vi "UHR-Fleezers Control (host) - 11.9b.vi"() -> ()   [LabVIEW 2014] (continued)
        n1961 = Or(x="Move to Position 5", y="Lower Ch. Cap.") -> (x .or. y?=w2805:bool)
        n1962 = Build Array("Move to Position 1", "Move to Position 2", "Move to Position 3", "Move to Position 4", w2805) -> (w2808:bool[])
        n1963 = Boolean Array To Number(Boolean array=w2808) -> (number=w2807:u32)
        n1964 = Logarithm Base 2(1:w2807) -> (0:w2806:dbl)
        n1965 = flat-sequence {
          tunnel: w2806 -> [w2817]
          tunnel: w2803 -> [w2815]
          tunnel: w2802 -> [w2814]
          frame #0 {
            n1966 = local read "Saved Stage Positions"() -> (w2825:dbl[][])
            n1967 = Array Subset(array=w2825, index (row)=w2817, length (row)=1 ("length"), index (col)=1 ("index"), length (col)=3 ("length")) -> (w2822:dbl[][])
            n1968 = Reshape Array(w2822, 3 ("dimension size")) -> (w2820:dbl[])
            n1969 = Array To Cluster(array=w2820) -> (cluster=w2819:cluster{"[0]":dbl, "[1]":dbl, "[2]":dbl})
            n1970 = call "Set Stage Position.vi"("Position"=w2819, "error in"=w2814, "VISA resource name in"=w2815) -> ("error out"=w2818:errorcluster)  [unwired: 2 out]
            n1971 = local write "Stage Moving"(TRUE ("Stage Moving")) -> ()
            n1972 = local write "Stage Control Serial Error"(w2818) -> ()
          }
          frame #1 {
            n1973 = local write "Stage Moving"(FALSE ("Stage Moving")) -> ()
            n1974 = call <vilib>:"Beep.vi"() -> ()  [unwired: 3 in, 9 out]
          }
        }
      }
      event "Set Current\nPos to 0,0,0": Value Change {
        # "DH is \"Define Home\""
        n1975 = event-data() -> ()  [unwired: 1 in, 6 out]
        n1976 = local write "Set Current\nPos to 0,0,0"(FALSE ("Set Current\nPos to 0,0,0")) -> ()
        n1977 = Concatenate Strings("1DH" ("string"), ";" ("string"), "2DH" ("string"), ";" ("string"), "3DH" ("string"), "\r") -> (w2833:string)
        n1978 = call-poly "VISA Configure Serial Port"("VISA resource name"=w2838, "baud rate (9600)"=u32 19200, "error in (no error)"=w2837) -> ("VISA resource name out"=w2835:refnum<visa-resource-name>, "error out"=w2834:errorcluster)  [unwired: 11 in]
        n1979 = VISA Write(VISA resource name=w2835, write buffer=w2833, error in (no error)=w2834) -> (error out=w2828:errorcluster)  [unwired: 2 out]
        n1980 = local write "Stage Control Serial Error"(w2828) -> ()
      }
      event "Got ADig bead": Value Change {
        n1981 = event-data() -> ()  [unwired: 1 in, 5 out]
        n1982 = flat-sequence {
          frame #0 {
            n1983 = local read "Cap 1 Samp Flow ON"() -> (w2843:bool)
            n1984 = case shown="True" w2843 {
              frame False {
              }
              frame True {
                n1985 = property on="Sample Channel\nFlow" class="Bool (strict)"("Val(Sgnl)"=TRUE ("Value (Signaling)")) -> ()  [unwired: 2 in, 2 out]
              }
            }
          }
          frame #1 {
            n1986 = property on="Inject Pump 3" class="Bool (strict)"("Val(Sgnl)"=FALSE ("Value (Signaling)")) -> ()  [unwired: 2 in, 2 out]
            n1987 = local write "Target"(FALSE ("Target")) -> ()
          }
          frame #2 {
            n1988 = property on="Move Cap. 1 (DNA Bottom)" class="Bool (strict)"("Val(Sgnl)"=TRUE ("Value (Signaling)")) -> ()  [unwired: 2 in, 2 out]
          }
        }
      }
      event "Force FB Script": Value Change {
        n1989 = event-data() -> ()  [unwired: 1 in, 5 out]
        n1990 = local write "Force FB Script"(FALSE ("Force FB Data\nScript")) -> ()
        n1991 = flat-sequence {
          tunnel: w2854 -> [w2858]
          tunnel: w2855 -> [w2859]
          tunnel: [w2859] -> w2850
          tunnel: [w2858] -> w2849
          tunnel: w2850 -> [w2862]
          tunnel: w2849 -> [w2861]
          tunnel: ["Trap Trig Fl."] -> w2851
          tunnel: [w2904] -> w2852
          tunnel: w2851 -> [w2904]
          tunnel: [w2908] -> w2853
          tunnel: w2852 -> [w2908]
          tunnel: w2853 -> [w2910]
          frame #0 {
            n1992 = property on="Trap D (MHz)" class="DigNum (strict)"("Val(Sgnl)"="Trap D Before Moving") -> ()  [unwired: 2 in, 2 out]
          }
          frame #1 {
            n1993 = local read "Saved Stage Positions"() -> (w2864:dbl[][])
            n1994 = local write "FB Trap Pos Offset"(0.0 ("FB Trap Pos Offset")) -> ()
            n1995 = property on="Trap Pos. FB Offset Factor" class="DigNum (strict)"("Val(Sgnl)"=i64 0 ("Value (Signaling)")) -> ()  [unwired: 2 in, 2 out]
            n1996 = local write "Stage Moving"(TRUE ("Stage Moving")) -> ()
            n1997 = call "move to saved stage position.vi"("error in"=w2861, "Stage VISA resource name in"=w2862, "Position"="Stage Position To Establish FB", "Saved Stage Positions"=w2864) -> ("error out"=w2860:errorcluster)  [unwired: 1 out]
            n1998 = local write "Stage Control Serial Error"(w2860) -> ()
          }
          frame #2 {
            n1999 = call <vilib>:"Beep.vi"("duration (msec)"=u32 100, "frequency (Hz)"=u32 20) -> ()  [unwired: 1 in, 9 out]
            n2000 = local write "Stage Moving"(FALSE ("Stage Moving")) -> ()
            n2001 = property on="Tab Control 2" class="TabCtl (strict)"("Val(Sgnl)"=T6."Feedback on Trap Position" ("Value (Signaling)")) -> ()  [unwired: 2 in, 2 out]
            n2002 = stacked-sequence {
              frame #0 {
                n2003 = Multiply(x="Wait (s)", y=u32 1000 ("milliseconds to wait")) -> (x*y=w2873:u32)
                n2004 = property on="Trap D (MHz)" class="DigNum (strict)"("Val(Sgnl)"="Starting Trap D (MHz)") -> ()  [unwired: 2 in, 2 out]
                n2005 = Wait (ms)(milliseconds to wait=w2873) -> ()  [unwired: 1 out]
              }
              frame #1 {
                n2006 = property on="Set Reading to\nSetpoint" class="Bool (strict)"("Val(Sgnl)"=TRUE ("Value (Signaling)")) -> ()  [unwired: 2 in, 2 out]
              }
            }
            n2007 = property on="Tab Control" class="TabCtl (strict)"("Val(Sgnl)"=T4."Trap Control (RF)" ("Value (Signaling)")) -> ()  [unwired: 2 in, 2 out]
          }
          frame #3 {
            n2008 = Wait (ms)(milliseconds to wait=u32 500) -> ()  [unwired: 1 out]
          }
          frame #4 {
            n2009 = property on="Trap Pos. FB ON" class="Bool (strict)"("Val(Sgnl)"=TRUE ("Value (Signaling)")) -> ()  [unwired: 2 in, 2 out]
            n2010 = Wait (ms)(milliseconds to wait=u32 250) -> ()  [unwired: 1 out]
          }
          frame #5 {
            n2011 = case shown="\"1\"" "Remove Action Offset Dropdown" {
              tunnel: TRUE ("Value (Signaling)") -> [w2885 w2893 w2901]
              frame "1" {
                n2012 = flat-sequence {
                  tunnel: w2885 -> [w2892]
                  frame #0 {
                    n2013 = local read "factor"() -> (w2887:dbl)
                    n2014 = Greater Than 0?(x=w2887) -> (x > 0?=w2891:bool)
                    n2015 = Select(t=1.0, s=w2891, f=-1.0) -> (s? t:f=w2888:dbl)
                    n2016 = Multiply(x=w2888, y=w2887) -> (x*y=w2886:dbl)
                    n2017 = local write "factor"(w2886) -> ()
                  }
                  frame #1 {
                    n2018 = property on="Remove Offset to factor" class="Bool (strict)"("Val(Sgnl)"=w2892) -> ()  [unwired: 2 in, 2 out]
                  }
                }
              }
              frame "2" {
                n2019 = flat-sequence {
                  tunnel: w2893 -> [w2900]
                  frame #0 {
                    n2020 = local read "factor"() -> (w2894:dbl)
                    n2021 = Greater Than 0?(x=w2894) -> (x > 0?=w2899:bool)
                    n2022 = Select(t=-1.0, s=w2899, f=1.0) -> (s? t:f=w2897:dbl)
                    n2023 = Multiply(x=w2894, y=w2897) -> (x*y=w2896:dbl)
                    n2024 = local write "factor"(w2896) -> ()
                  }
                  frame #1 {
                    n2025 = property on="Remove Offset to factor" class="Bool (strict)"("Val(Sgnl)"=w2900) -> ()  [unwired: 2 in, 2 out]
                  }
                }
              }
              frame "0", Default {
                n2026 = property on="Remove Action Offset" class="Bool (strict)"("Val(Sgnl)"=w2901) -> ()  [unwired: 2 in, 2 out]
              }
            }
            n2027 = case shown="False" "Trap Trig Fl." {
              frame False {
                n2028 = case shown="True" "Green ON after FB ON?" {
                  selector: "Green ON after FB ON?" -> [_ w2903]
                  frame False {
                  }
                  frame True {
                    n2029 = property on="Green ON/Interlacing" class="Bool (strict)"("Val(Sgnl)"=w2903) -> ()  [unwired: 2 in, 2 out]
                  }
                }
              }
              frame True {
              }
            }
            n2030 = Wait (ms)(milliseconds to wait=u32 250) -> ()  [unwired: 1 out]
          }
          frame #6 {
            n2031 = property on="Start Saving" class="Bool (strict)"("Val(Sgnl)"=TRUE ("Value (Signaling)")) -> ()  [unwired: 2 in, 2 out]
            n2032 = Wait (ms)(milliseconds to wait=u32 5000) -> ()  [unwired: 1 out]
          }
          frame #7 {
            w2907 = TRUE ("Value (Signaling)")
            n2033 = property on="Rem fb disp offset" class="Bool (strict)"("Val(Sgnl)"=w2907) -> ()  [unwired: 2 in, 2 out]
            n2034 = property on="Remove Offset" class="Bool (strict)"("Val(Sgnl)"=w2907) -> ()  [unwired: 2 in, 2 out]
            n2035 = Wait (ms)(milliseconds to wait=u32 100) -> ()  [unwired: 1 out]
          }
          frame #8 {
            n2036 = case shown="True" w2910 {
              frame False {
              }
              frame True {
                n2037 = local write "Trap Trig. Fl."(TRUE ("Value (Signaling)")) -> ()
              }
            }
          }
          frame #9 {
            n2038 = local read "Tether"() -> (w2913:bool)
            n2039 = And(x="Start dipping after?", y=w2913) -> (x .and. y?=w2912:bool)
            n2040 = case shown="True" w2912 {
              frame False {
              }
              frame True {
                n2041 = flat-sequence {
                  frame #0 {
                    n2042 = Multiply(x="Delay before dipping (s)", y=1000.0) -> (x*y=w2916:dbl)
                    n2043 = Wait (ms)(milliseconds to wait=w2916) -> ()  [unwired: 1 out]
                  }
                  frame #1 {
                    n2044 = property on="Dip for Protein" class="Bool (strict)"("Val(Sgnl)"=TRUE ("Value (Signaling)")) -> ()  [unwired: 2 in, 2 out]
                    n2045 = local write "Scripts"(T29."Dipping") -> ()
                  }
                }
              }
            }
          }
        }
      }
      event "Rupture Script": Value Change {
        n2046 = event-data() -> ()  [unwired: 1 in, 5 out]
        n2047 = local write "Rupture Script"(FALSE ("Rupture Script")) -> ()
        n2048 = flat-sequence {
          frame #0 {
            w2922 = TRUE
            w2927 = FALSE
            # "Number 6 for now is the\nrupture-experiment\nparameters."
            n2049 = local read "Starting Trap D (MHz)"() -> (w2928:dbl)
            n2050 = local write "Restart DMA? (AOD)"(w2927) -> ()
            n2051 = Replace Array Subset(array=u32[] [0] ("Index Values"), new element=6, index=0) -> (w2923:u32[])
            n2052 = local write "Save scans"(w2927) -> ()
            n2053 = property on="Trap D (MHz)" class="DigNum (strict)"("Val(Sgnl)"=w2928) -> ()  [unwired: 2 in, 2 out]
            n2054 = property on="Saved AOD Raster Scan Parameter Sets" class="Arr (strict)"("Index Values"=w2923) -> ()  [unwired: 2 in, 2 out]
            n2055 = property on="Start Saving" class="Bool (strict)"("Val(Sgnl)"=w2922) -> ()  [unwired: 2 in, 2 out]
            n2056 = property on="Green ON/Interlacing" class="Bool (strict)"("Val(Sgnl)"=w2922) -> ()  [unwired: 2 in, 2 out]
          }
          frame #1 {
            n2057 = property on="Load parameters" class="Bool (strict)"("Val(Sgnl)"=TRUE ("Value (Signaling)")) -> ()  [unwired: 2 in, 2 out]
          }
        }
      }
      event "Fixed Traps Script": Value Change {
        n2058 = event-data() -> ()  [unwired: 1 in, 5 out]
        n2059 = local write "Fixed Traps Script"(FALSE ("Fixed Traps Data\nScript")) -> ()
        n2060 = flat-sequence {
          frame #0 {
            n2061 = case shown="True" "Green ON" {
              frame False {
              }
              frame True {
                n2062 = property on="Green ON/Interlacing" class="Bool (strict)"("Val(Sgnl)"=TRUE) -> ()  [unwired: 2 in, 2 out]
              }
            }
            n2063 = local write "Offset (nm)"(0.0 ("Offset (nm)")) -> ()
            n2064 = property on="Sample Channel\nFlow" class="Bool (strict)"("Val(Sgnl)"=FALSE ("Value (Signaling)")) -> ()  [unwired: 2 in, 2 out]
            n2065 = property on="Trap D (MHz)" class="DigNum (strict)"("Val(Sgnl)"="Fixed Traps Trap Delta (MHz)") -> ()  [unwired: 2 in, 2 out]
          }
          frame #1 {
            n2066 = Wait (ms)(milliseconds to wait=u32 1000) -> ()  [unwired: 1 out]
          }
          frame #2 {
            n2067 = local write "Start Saving"(TRUE ("Start Saving")) -> ()
          }
          frame #3 {
            n2068 = local read "Bead Sep. Int. Time (s)"() -> (w2938:dbl)
            n2069 = Multiply(x=w2938, y=1000.0) -> (x*y=w2940:dbl)
            n2070 = Wait (ms)(milliseconds to wait=w2940) -> ()  [unwired: 1 out]
          }
          frame #4 {
            n2071 = property on="Remove Offset" class="Bool (strict)"("Val(Sgnl)"=TRUE ("Value (Signaling)")) -> ()  [unwired: 2 in, 2 out]
          }
          frame #5 {
            n2072 = property on="Dip for Protein" class="Bool (strict)"("Val(Sgnl)"="Start dipping after?") -> ()  [unwired: 2 in, 2 out]
          }
        }
      }
      event "Got DNA bead": Value Change {
        n2073 = event-data() -> ()  [unwired: 1 in, 5 out]
        n2074 = flat-sequence {
          frame #0 {
            n2075 = local read "Daq spot flow on"() -> (w2945:bool)
            n2076 = case shown="True" w2945 {
              frame False {
              }
              frame True {
                n2077 = property on="Sample Channel\nFlow" class="Bool (strict)"("Val(Sgnl)"=TRUE ("Value (Signaling)")) -> ()  [unwired: 2 in, 2 out]
              }
            }
            n2078 = property on="Got DNA bead" class="Bool"("Key Focus"=FALSE) -> ()  [unwired: 2 in, 2 out]
          }
          frame #1 {
            n2079 = property on="Inject Pump 1" class="Bool (strict)"("Val(Sgnl)"=FALSE ("Value (Signaling)")) -> ()  [unwired: 2 in, 2 out]
          }
          frame #2 {
            n2080 = property on="Cal/Data Acq. Spot" class="Bool (strict)"("Val(Sgnl)"=TRUE ("Value (Signaling)")) -> ()  [unwired: 2 in, 2 out]
          }
        }
      }
      event "Take Stepping Data": Value Change {
        n2081 = event-data() -> ()  [unwired: 1 in, 5 out]
        n2082 = local read "Save ave N"() -> (w2957:dbl)
        n2083 = flat-sequence {
          tunnel: w2957 -> [w2959]
          tunnel: [w2959] -> w2952
          tunnel: [w2961] -> w2953
          tunnel: w2952 -> [w2961]
          tunnel: [w2963] -> w2954
          tunnel: w2953 -> [w2963]
          tunnel: [w2966] -> w2955
          tunnel: w2954 -> [w2966]
          tunnel: [w2968] -> w2956
          tunnel: w2955 -> [w2968]
          tunnel: [w2970] -> w2950
          tunnel: w2956 -> [w2970]
          tunnel: w2950 -> [w2973]
          tunnel: [w2973] -> w2949
          tunnel: w2949 -> [w2974]
          tunnel: [w2974] -> w2951
          tunnel: w2951 -> [w2980]
          frame #0 {
            n2084 = property on="Save ave N" class="DigNum (strict)"("Val(Sgnl)"="Save ave factor") -> ()  [unwired: 2 in, 2 out]
          }
          frame #1 {
            n2085 = Wait (ms)(milliseconds to wait=u32 100) -> ()  [unwired: 1 out]
          }
          frame #2 {
            n2086 = local read "Offset 2 Start (MHz)"() -> (w2965:dbl)
            n2087 = property on="Saved AOD Raster Scan Parameter Sets" class="Arr (strict)"("Index Values"=u32[] [2]) -> ()  [unwired: 2 in, 2 out]
            n2088 = property on="Trap D (MHz)" class="DigNum (strict)"("Val(Sgnl)"=w2965) -> ()  [unwired: 2 in, 2 out]
          }
          frame #3 {
            n2089 = property on="Load parameters" class="Bool (strict)"("Val(Sgnl)"=TRUE ("Value (Signaling)")) -> ()  [unwired: 2 in, 2 out]
          }
          frame #4 {
            n2090 = Wait (ms)(milliseconds to wait=u32 100) -> ()  [unwired: 1 out]
          }
          frame #5 {
            n2091 = property on="Trap Raster Scan" class="Bool (strict)"("Val(Sgnl)"=TRUE ("Value (Signaling)")) -> ()  [unwired: 2 in, 2 out]
          }
          frame #6 {
            n2092 = Wait (ms)(milliseconds to wait=u32 1000) -> ()  [unwired: 1 out]
          }
          frame #7 {
            n2093 = while {
              stop <- w2977 stop-if-true
              n2094 = local read "Raster Scanning..."() -> (w2979:bool)
              n2095 = local read "Saving..."() -> (w2978:bool)
              n2096 = Not(x=w2978) -> (.not. x?=w2975:bool)
              n2097 = Not(x=w2979) -> (.not. x?=w2976:bool)
              n2098 = And(x=w2976, y=w2975) -> (x .and. y?=w2977:bool)
            }
          }
          frame #8 {
            n2099 = property on="Save ave N" class="DigNum (strict)"("Val(Sgnl)"=w2980) -> ()  [unwired: 2 in, 2 out]
          }
        }
      }
      event "Step Size (nm)": Value Change {
        n2100 = event-data() -> ()  [unwired: 1 in, 5 out]
        n2101 = flat-sequence {
          frame #0 {
            n2102 = property on="Saved AOD Raster Scan Parameter Sets" class="Arr (strict)"("Index Values"=u32[] [1]) -> ()  [unwired: 2 in, 2 out]
          }
          frame #1 {
            n2103 = Multiply(x="N Steps", y="Step Size (nm)") -> (x*y=w2982:dbl)
            n2104 = property on="Scan Speed AOD (nm/s) 2" class="DigNum (strict)"("Value"="Step Size (nm)") -> ()  [unwired: 2 in, 2 out]
            n2105 = property on="Step Size AOD (nm) 2" class="DigNum (strict)"("Value"="Step Size (nm)") -> ()  [unwired: 2 in, 2 out]
            n2106 = property on="Scan Range AOD (nm) 2" class="DigNum (strict)"("Value"=w2982) -> ()  [unwired: 2 in, 2 out]
          }
        }
      }
      event "Take Detection Laser\nImage": Value Change {
        n2107 = event-data() -> ()  [unwired: 1 in, 5 out]
        n2108 = flat-sequence {
          tunnel: [w3010] -> w3000
          tunnel: [w3009] -> w2993
          tunnel: [w3008] -> w2985
          tunnel: [w3013] -> w3001
          tunnel: w3000 -> [w3013]
          tunnel: [w3012] -> w2994
          tunnel: w2993 -> [w3012]
          tunnel: [w3011] -> w2986
          tunnel: w2985 -> [w3011]
          tunnel: [w3017] -> w3002
          tunnel: w3001 -> [w3017]
          tunnel: [w3016] -> w2995
          tunnel: w2994 -> [w3016]
          tunnel: [w3015] -> w2987
          tunnel: w2986 -> [w3015]
          tunnel: [w3023] -> w3003
          tunnel: w3002 -> [w3023]
          tunnel: [w3022] -> w2996
          tunnel: w2995 -> [w3022]
          tunnel: [w3021] -> w2988
          tunnel: w2987 -> [w3021]
          tunnel: [w3027] -> w3004
          tunnel: w3003 -> [w3027]
          tunnel: [w3026] -> w2997
          tunnel: w2996 -> [w3026]
          tunnel: [w3025] -> w2989
          tunnel: w2988 -> [w3025]
          tunnel: [w3031] -> w3005
          tunnel: w3004 -> [w3031]
          tunnel: [w3030] -> w2998
          tunnel: w2997 -> [w3030]
          tunnel: [w3029] -> w2990
          tunnel: w2989 -> [w3029]
          tunnel: [w3035] -> w3006
          tunnel: w3005 -> [w3035]
          tunnel: [w3034] -> w2999
          tunnel: w2998 -> [w3034]
          tunnel: [w3033] -> w2991
          tunnel: w2990 -> [w3033]
          tunnel: w3006 -> [w3041]
          tunnel: w2999 -> [w3040]
          tunnel: [w3038] -> w2992
          tunnel: w2991 -> [w3038]
          tunnel: w2992 -> [w3042]
          frame #0 {
            n2109 = local read "Green ON/Interlacing"() -> (w3010:bool)
            n2110 = local read "Green laser mode"() -> (w3009:enum32{"Laser ON", "Laser OFF", "Interlace"})
            n2111 = local read "Green FB On/Off"() -> (w3008:bool)
          }
          frame #1 {
            n2112 = property on="Green FB On/Off" class="Bool (strict)"("Val(Sgnl)"=FALSE ("Value (Signaling)")) -> ()  [unwired: 2 in, 2 out]
          }
          frame #2 {
            n2113 = property on="Green ON/Interlacing" class="Bool (strict)"("Val(Sgnl)"=TRUE ("Value (Signaling)")) -> ()  [unwired: 2 in, 2 out]
            n2114 = property on="Flip Green Filter" class="Bool (strict)"("Val(Sgnl)"=TRUE ("Value (Signaling)")) -> ()  [unwired: 2 in, 2 out]
            n2115 = property on="Green laser mode" class="RadioBtnsControl (strict)"("Val(Sgnl)"=enum32{"Laser ON", "Laser OFF", "Interlace"}."Laser ON" ("Value (Signaling)")) -> ()  [unwired: 2 in, 2 out]
          }
          frame #3 {
            n2116 = Wait (ms)(milliseconds to wait=u32 500) -> ()  [unwired: 1 out]
          }
          frame #4 {
            n2117 = property on="Confocal\nImage" class="Bool (strict)"("Val(Sgnl)"=TRUE ("Value (Signaling)")) -> ()  [unwired: 2 in, 2 out]
          }
          frame #5 {
            n2118 = Wait (ms)(milliseconds to wait=u32 2000) -> ()  [unwired: 1 out]
          }
          frame #6 {
            n2119 = while {
              stop <- w3036 stop-if-true
              n2120 = local read "Saving..."() -> (w3037:bool)
              n2121 = Not(x=w3037) -> (.not. x?=w3036:bool)
            }
          }
          frame #7 {
            n2122 = property on="Flip Green Filter" class="Bool (strict)"("Val(Sgnl)"=TRUE ("Value (Signaling)")) -> ()  [unwired: 2 in, 2 out]
            n2123 = property on="Green ON/Interlacing" class="Bool (strict)"("Val(Sgnl)"=w3041) -> ()  [unwired: 2 in, 2 out]
            n2124 = property on="Green laser mode" class="RadioBtnsControl (strict)"("Val(Sgnl)"=w3040) -> ()  [unwired: 2 in, 2 out]
          }
          frame #8 {
            n2125 = property on="Green FB On/Off" class="Bool (strict)"("Val(Sgnl)"=w3042) -> ()  [unwired: 2 in, 2 out]
          }
        }
      }
      event "Stop All": Value Change {
        n2126 = event-data() -> ()  [unwired: 1 in, 5 out]
        n2127 = local read "Stop All"() -> (w3043:bool)
      }
    }
    n2128 = node-c288() -> ()  [unwired: 1 in, 1 out]
  }
  n2129 = node-c288() -> (w115:T21)  [unwired: 4 out]
  n2130 = timed-loop "Mouse control: trap position (AOM deflection), set confocal spot from image" {
    tunnel: [w3045] -> w203
    tunnel: w23 -> [w3044]
    timing: w115 -> [_]
    timing-out: [_] -> w114
    stop <- w3045 stop-if-true
    n2131 = node-c288() -> ()  [unwired: 2 out]
    n2132 = event shown="[0] \"Pane\": Mouse Down" {
      selector: _ -> [_ _]
      dyn-events: _ -> [_ _]
      timeout: _ -> [_ _]
      tunnel: w3044 -> [w3048 _]
      event Mouse Down {
        n2133 = event-data() -> ("Time"=w3050:u32, "Coords"=w3049:T7, "Button"=w3051:u16)  [unwired: 6 out]
        n2134 = case shown="1" w3051 {
          tunnel: w3050 -> [_ _ w3190]
          tunnel: w3049 -> [_ w3056 w3188]
          tunnel: w3048 -> [_ _ w3186]
          frame 0, Default {
          }
          frame 1 {
            n2135 = property on="APD 2" class="ImageControl"() -> ("Displayed Image Position"=w3070:cluster{"Left":i32, "Top":i32})  [unwired: 2 in, 2 out]
            n2136 = control-ref of="Primary Video Display"() -> (w3063:refnum<vi>)
            n2137 = property on="APD 1" class="ImageControl"() -> ("Displayed Image Position"=w3099:cluster{"Left":i32, "Top":i32})  [unwired: 2 in, 2 out]
            n2138 = property on="Detection Laser X" class="ImageControl"() -> ("Displayed Image Position"=w3096:cluster{"Left":i32, "Top":i32})  [unwired: 2 in, 2 out]
            n2139 = property on="Detection Laser Y" class="ImageControl"() -> ("Displayed Image Position"=w3095:cluster{"Left":i32, "Top":i32})  [unwired: 2 in, 2 out]
            n2140 = property on="APD 2" class="ImageControl"() -> ("Displayed Image Size"=w3069:cluster{"Width":u32, "Height":u32})  [unwired: 2 in, 2 out]
            n2141 = property on="APD 1" class="ImageControl"() -> ("Displayed Image Size"=w3097:cluster{"Width":u32, "Height":u32})  [unwired: 2 in, 2 out]
            n2142 = property on="Detection Laser X" class="ImageControl"() -> ("Displayed Image Size"=w3098:cluster{"Width":u32, "Height":u32})  [unwired: 2 in, 2 out]
            n2143 = property on="Detection Laser Y" class="ImageControl"() -> ("Displayed Image Size"=w3094:cluster{"Width":u32, "Height":u32})  [unwired: 2 in, 2 out]
            n2144 = property class="ImageControl"(reference=w3063) -> ("Displayed Image Position"=w3061:cluster{"Left":i32, "Top":i32})  [unwired: 1 in, 2 out]
            n2145 = property class="ImageControl"(reference=w3063) -> ("Displayed Image Size"=w3062:cluster{"Width":u32, "Height":u32})  [unwired: 1 in, 2 out]
            n2146 = Unbundle By Name(w3069) -> ("Width"=w3066:u32, "Height"=w3065:u32)
            n2147 = Unbundle By Name(w3070) -> ("Left"=w3068:i32, "Top"=w3067:i32)
            n2148 = Unbundle By Name(w3097) -> ("Width"=w3091:u32, "Height"=w3090:u32)
            n2149 = Unbundle By Name(w3098) -> ("Width"=w3087:u32, "Height"=w3086:u32)
            n2150 = Unbundle By Name(w3094) -> ("Width"=w3083:u32, "Height"=w3082:u32)
            n2151 = Unbundle By Name(w3099) -> ("Left"=w3093:i32, "Top"=w3092:i32)
            n2152 = Unbundle By Name(w3096) -> ("Left"=w3089:i32, "Top"=w3088:i32)
            n2153 = Unbundle By Name(w3095) -> ("Left"=w3085:i32, "Top"=w3084:i32)
            n2154 = Bundle("Left"=w3068, "Top"=w3067, "Width"=w3066, "Height"=w3065) -> (w3064:T30)  [unwired: 1 in]
            n2155 = Bundle("Left"=w3093, "Top"=w3092, "Width"=w3091, "Height"=w3090) -> (w3081:T30)  [unwired: 1 in]
            n2156 = Bundle("Left"=w3089, "Top"=w3088, "Width"=w3087, "Height"=w3086) -> (w3080:T30)  [unwired: 1 in]
            n2157 = Bundle("Left"=w3085, "Top"=w3084, "Width"=w3083, "Height"=w3082) -> (w3079:T30)  [unwired: 1 in]
            n2158 = Unbundle By Name(w3062) -> ("Width"=w3058:u32, "Height"=w3057:u32)
            n2159 = Unbundle By Name(w3061) -> ("Left"=w3060:i32, "Top"=w3059:i32)
            n2160 = Build Cluster Array(w3064, w3081, w3080, w3079) -> (w3078:T31)
            n2161 = Bundle("Left"=w3060, "Top"=w3059, "Width"=w3058, "Height"=w3057) -> (w3053:T30)  [unwired: 1 in]
            n2162 = for {
              tunnel: w3056 -> [w3132]
              tunnel: w3078 -> [w3133] mode=indexing
              shift-right: [w3130] -> w3076
              shift-left: TRUE -> [w3131]
              shift-right: [w3129] -> w3074
              shift-left: _ -> [w3125]
              shift-right: [w3128] -> w3073
              shift-left: _ -> [w3124]
              shift-right: [w3127] -> w3072
              shift-left: _ -> [w3123]
              shift-right: [w3126] -> w3071
              shift-left: _ -> [w3122]
              n2163 = case shown="True" w3131 {
                selector: w3131 -> [w3138 _]
                tunnel: w3133 -> [_ w3147]
                tunnel: w3132 -> [_ w3145]
                tunnel: [w3138 w3143] -> w3130
                tunnel: [w3137 w3142] -> w3129
                tunnel: [w3136 w3141] -> w3128
                tunnel: [w3135 w3140] -> w3127
                tunnel: [w3134 w3139] -> w3126
                tunnel: w3125 -> [w3137 _]
                tunnel: w3124 -> [w3136 _]
                tunnel: w3123 -> [w3135 _]
                tunnel: w3122 -> [w3134 _]
                frame False {
                }
                frame True {
                  n2164 = Unbundle(w3147) -> (w3146:T30)
                  n2165 = call "isclickinwindow.vi"("Image Param"=w3146, "Point32"=w3145) -> ("4 Y"=w3139:i32, "3 Height"=w3140:i32, "2 X"=w3141:i32, "1 Width"=w3142:i32, "In image?"=w3144:bool)  [unwired: 1 in]
                  n2166 = Not(x=w3144) -> (.not. x?=w3143:bool)
                }
              }
            }
            n2167 = call "isclickinwindow.vi"("Image Param"=w3053, "Point32"=w3056) -> ("4 Y"=w3054:i32, "2 X"=w3055:i32, "In image?"=w3052:bool)  [unwired: 1 in, 2 out]
            n2168 = case shown="True" w3052 {
              tunnel: w3055 -> [_ w3103]
              tunnel: w3054 -> [_ w3106]
              frame False {
              }
              frame True {
                w3115 = 2
                n2169 = Subtract(x=480, y=w3106) -> (x-y=w3105:i32)
                n2170 = Unbundle("Target size") -> ("Width"=w3116:dbl, "Height"=w3114:dbl)
                n2171 = Subtract(x=w3103, y=2) -> (x-y=w3102:i32)
                n2172 = Divide(x=w3114, y=w3115) -> (x/y=w3112:dbl)
                n2173 = Divide(x=w3116, y=w3115) -> (x/y=w3113:dbl)
                n2174 = Subtract(x=w3102, y=w3113) -> (x-y=w3111:dbl)
                n2175 = Add(x=w3102, y=w3113) -> (x+y=w3109:dbl)
                n2176 = Subtract(x=w3105, y=w3112) -> (x-y=w3110:dbl)
                n2177 = Add(x=w3105, y=w3112) -> (x+y=w3108:dbl)
                n2178 = Bundle(w3102, w3105) -> (w3118:cluster{i32, i32})  [unwired: 1 in]
                n2179 = Bundle(w3111, w3110, w3109, w3108) -> (w3100:cluster{dbl, dbl, dbl, dbl})  [unwired: 1 in]
                n2180 = case shown="True" "Set target" {
                  tunnel: w3118 -> [_ w3121]
                  tunnel: w3100 -> [_ w3119]
                  frame False {
                  }
                  frame True {
                    n2181 = local write "Target coordinates"(w3119) -> ()
                    n2182 = local write "Set target"(FALSE ("Set target")) -> ()
                    "Video coordinates" <- w3121
                  }
                }
              }
            }
            n2183 = Not(x=w3076) -> (.not. x?=w3075:bool)
            n2184 = case shown="True" w3075 {
              tunnel: w3073 -> [_ w3161]
              tunnel: w3071 -> [_ w3160]
              tunnel: w3074 -> [_ w3159]
              tunnel: w3072 -> [_ w3158]
              frame False {
              }
              frame True {
                w3148 = FALSE ("Get Point")
                n2185 = local read "Scan lines (y)"() -> (w3163:u64)
                n2186 = disable-structure shown="Disabled" {
                  frame Disabled {
                  }
                  frame Enabled {
                  }
                }
                n2187 = local read "Actual MCL Inc (V)"() -> (w3157:dbl)
                n2188 = local read "Scan steps (MCL)"() -> (w3162:u64)
                n2189 = Divide "Y Pix/step"(x=w3158, y=w3163) -> (x/y=w3170:dbl)
                n2190 = Divide "Y V/pix"(x=w3157, y=w3170) -> (x/y=w3169:dbl)
                n2191 = Divide "Y half step offset"(x=w3157, y=2.0) -> (x/y=w3171:dbl)
                n2192 = Divide "X pix/step"(x=w3159, y=w3162) -> (x/y=w3168:dbl)
                n2193 = Negate(x=w3171) -> (-x=w3172:dbl)
                n2194 = local read "Initial Y"() -> (w3178:dbl)
                n2195 = Multiply(x=w3160, y=w3169) -> (x*y=w3179:dbl)
                n2196 = Divide "X half step offset"(x=w3157, y=2.0) -> (x/y=w3165:dbl)
                n2197 = Divide "X V/pix"(x=w3157, y=w3168) -> (x/y=w3167:dbl)
                n2198 = Multiply(x=w3157, y=w3162) -> (x*y=w3174:dbl)
                n2199 = Compound Arithmetic op=ADD(w3172, w3179, w3178) -> (w3149:dbl)
                "Pointer Y (V)" <- w3149
                n2200 = Multiply(x=w3167, y=w3161) -> (x*y=w3176:dbl)
                n2201 = Negate(x=w3165) -> (-x=w3164:dbl)
                n2202 = local read "Initial X"() -> (w3177:dbl)
                n2203 = Negate(x=w3176) -> (-x=w3175:dbl)
                n2204 = Compound Arithmetic op=ADD(w3164, w3174, w3177, w3175) -> (w3150:dbl)
                "Pointer X (V)" <- w3150
                n2205 = case shown="True" "Set High F Confocal Spot (X-Y)" {
                  tunnel: w3150 -> [_ w3180]
                  tunnel: w3149 -> [_ w3181]
                  frame False {
                  }
                  frame True {
                    "Confocal Y 2 (V)" <- w3181
                    "Confocal X 2 (V)" <- w3180
                  }
                }
                n2206 = Or(x="Set X Only", y="Set Confocal Spot (X-Y)") -> (x .or. y?=w3153:bool)
                n2207 = Or(x="Set Confocal Spot (X-Y)", y="Set Y Only") -> (x .or. y?=w3152:bool)
                n2208 = case shown="True" w3153 {
                  tunnel: w3150 -> [_ w3182]
                  frame False {
                  }
                  frame True {
                    n2209 = property on="AO2" class="Slide (strict)"("Val(Sgnl)"=w3182) -> ()  [unwired: 2 in, 2 out]
                    "Confocal X 1 (V)" <- w3182
                  }
                }
                n2210 = case shown="True" w3152 {
                  tunnel: w3149 -> [_ w3183]
                  frame False {
                  }
                  frame True {
                    n2211 = property on="AO1" class="Slide (strict)"("Val(Sgnl)"=w3183) -> ()  [unwired: 2 in, 2 out]
                    "Confocal Y 1 (V)" <- w3183
                  }
                }
                n2212 = local write "Set High F Confocal Spot (X-Y)"(w3148) -> ()
                n2213 = local write "Set Confocal Spot (X-Y)"(w3148) -> ()
                n2214 = local write "Set X Only"(w3148) -> ()
                n2215 = local write "Set Y Only"(w3148) -> ()
              }
            }
          }
          frame 3 {
            n2216 = local read "BD 2 Frequency 1 (MHz)"() -> (w3184:dbl)
            n2217 = local read "BD 1 Frequency 1 (MHz)"() -> (w3185:dbl)
            n2218 = local write "Manipulating Trap"(TRUE ("Manipulating Trap")) -> ()
            n2219 = local write "Coords"(T7 {"Horizontal"=0, "Vertical"=0} ("Coords")) -> ()
            n2220 = while {
              tunnel: w3190 -> [w3195]
              tunnel: w3188 -> [w3194]
              tunnel: w3186 -> [w3193]
              tunnel: w3185 -> [w3192]
              tunnel: w3184 -> [w3191]
              stop <- w3196 stop-if-true
              n2221 = event shown="[0] \"Pane\": Mouse Move" {
                selector: _ -> [_ _]
                dyn-events: _ -> [_ _]
                timeout: _ -> [_ _]
                tunnel: ["Force Manip Abort" w3260] -> w3196
                tunnel: w3195 -> [w3203 _]
                tunnel: w3194 -> [w3201 _]
                tunnel: w3193 -> [w3200 _]
                tunnel: w3192 -> [w3199 _]
                tunnel: w3191 -> [w3198 _]
                event Mouse Move {
                  n2222 = event-data() -> ("Time"=w3204:u32, "Coords"=w3205:T7)  [unwired: 3 out]
                  n2223 = Less?(x=w3204, y=w3203) -> (x < y?=w3202:bool)
                  n2224 = case "Makes sure old motion events prior to mouse click aren't used" shown="False" w3202 {
                    tunnel: w3205 -> [w3247 _]
                    tunnel: w3201 -> [w3248 _]
                    tunnel: w3200 -> [w3225 _]
                    tunnel: w3199 -> [w3221 _]
                    tunnel: w3198 -> [w3220 _]
                    frame False {
                      n2225 = Subtract(x=w3247, y=w3248) -> (x-y=w3246:T7)
                      "Coords" <- w3246
                      n2226 = local read "Y RF Frequency Limits (MHz)"() -> (w3206:T16)
                      n2227 = To Double Precision Float(number=w3246) -> (double precision float=w3245:cluster{"Horizontal":dbl, "Vertical":dbl})
                      n2228 = Multiply(x=cluster{"Horizontal":dbl, "Vertical":dbl} {"Horizontal"=-1.0, "Vertical"=1.0}, y="Manipulation Scaling") -> (x*y=w3241:cluster{"Horizontal":dbl, "Vertical":dbl})
                      n2229 = local read "X RF Frequency Limits (MHz)"() -> (w3207:T16)
                      n2230 = Multiply(x=w3245, y=w3241) -> (x*y=w3243:cluster{"Horizontal":dbl, "Vertical":dbl})
                      n2231 = Unbundle By Name(w3243) -> ("Horizontal"=w3238:dbl, "Vertical"=w3242:dbl)
                      n2232 = Unbundle By Name(w3206) -> ("Maximum"=w3209:dbl, "Minimum"=w3208:dbl)
                      n2233 = Boolean To (0,1)(Boolean="Manip. X?") -> (0, 1=w3236:i16)
                      n2234 = Boolean To (0,1)(Boolean="Manip. Y?") -> (0, 1=w3233:i16)
                      n2235 = local read "BD 1 Frequency 2 (MHz)"() -> (w3223:dbl)
                      n2236 = Multiply(x=w3242, y=w3233) -> (x*y=w3235:dbl)
                      n2237 = Multiply(x=w3236, y=w3238) -> (x*y=w3239:dbl)
                      n2238 = local read "BD 2 Frequency 2 (MHz)"() -> (w3222:dbl)
                      n2239 = Unbundle By Name(w3207) -> ("Maximum"=w3211:dbl, "Minimum"=w3210:dbl)
                      n2240 = Add(x=w3220, y=w3235) -> (x+y=w3213:dbl)
                      n2241 = Add(x=w3221, y=w3239) -> (x+y=w3215:dbl)
                      n2242 = In Range and Coerce(upper limit=w3211, x=w3215, lower limit=w3210) -> (coerced(x)=w3214:dbl)  [unwired: 1 out]
                      n2243 = In Range and Coerce(upper limit=w3209, x=w3213, lower limit=w3208) -> (coerced(x)=w3212:dbl)  [unwired: 1 out]
                      n2244 = Subtract(x=w3214, y=w3223) -> (x-y=w3232:dbl)
                      n2245 = Subtract(x=w3212, y=w3222) -> (x-y=w3231:dbl)
                      n2246 = Square(x=w3232) -> (x^2=w3230:dbl)
                      n2247 = Square(x=w3231) -> (x^2=w3229:dbl)
                      n2248 = Add(x=w3230, y=w3229) -> (x+y=w3228:dbl)
                      n2249 = Square Root(x=w3228) -> (sqrt(x)=w3224:dbl)
                      n2250 = In Range and Coerce(upper limit="Limit Max (MHz)", x=w3224, lower limit="Limit Min (MHz)") -> (In Range?=w3217:bool)  [unwired: 1 out]
                      n2251 = Not(x="Limits Enable") -> (.not. x?=w3216:bool)
                      n2252 = Or(x=w3217, y=w3216) -> (x .or. y?=w3218:bool)
                      n2253 = case shown="True" w3218 {
                        tunnel: w3225 -> [_ w3258]
                        tunnel: w3224 -> [_ w3249]
                        tunnel: w3214 -> [_ w3256]
                        tunnel: w3223 -> [_ w3255]
                        tunnel: w3212 -> [_ w3254]
                        tunnel: w3222 -> [_ w3253]
                        tunnel: w3207 -> [_ w3251]
                        tunnel: w3206 -> [_ w3250]
                        frame False {
                        }
                        frame True {
                          n2254 = local read "BD 1 Frequency 3 (MHz)"() -> (w3257:dbl)
                          n2255 = local read "BD 2 Frequency 3 (MHz)"() -> (w3252:dbl)
                          n2256 = local write "Trap D (MHz)"(w3249) -> ()
                          n2257 = call "set RF board frequency - interlace.vi"("Board 2 Frequency Limits"=w3250, "Board 1 Frequency Limits"=w3251, "FPGA VI Reference In"=w3258, "Board 2 Frequency 3 (MHz)"=w3252, "Board 1 Frequency 3 (MHz)"=w3257, "Board 2 Frequency 2 (MHz)"=w3253, "Board 2 Frequency 1 (MHz)"=w3254, "Board 1 Frequency 2 (MHz)"=w3255, "Board 1 Frequency 1  (MHz)"=w3256) -> ()  [unwired: 1 in, 2 out]
                          n2258 = local write "BD 2 Frequency 1 (MHz)"(w3254) -> ()
                          n2259 = local write "BD 1 Frequency 1 (MHz)"(w3256) -> ()
                        }
                      }
                    }
                    frame True {
                    }
                  }
                }
                event Mouse Up {
                  n2260 = event-data() -> ("Button"=w3259:u16)  [unwired: 8 out]
                  n2261 = case shown="3" w3259 {
                    tunnel: [FALSE TRUE] -> w3260
                    frame 0, Default {
                    }
                    frame 3 {
                      n2262 = local read "Trap D (MHz)"() -> (w3262:dbl)
                      n2263 = property on="Initial D (MHz)" class="DigNum (strict)"("Val(Sgnl)"=w3262) -> ()  [unwired: 2 in, 2 out]
                      n2264 = local write "Manipulating Trap"(FALSE ("Manipulating Trap")) -> ()
                    }
                  }
                }
              }
            }
          }
        }
      }
      event Mouse Move {
        n2265 = event-data() -> ()  [unwired: 6 out]
      }
    }
    n2266 = local read "Stop All"() -> (w3045:bool)
    n2267 = node-c288() -> ()  [unwired: 2 out]
  }
  n2268 = node-c288(w112) -> ()  [unwired: 1 out]
  n2269 = node-c288(w114) -> ()  [unwired: 1 out]
  n2270 = node-c288(w100) -> ()  [unwired: 1 out]
  n2271 = flat-sequence "Video" {
    tunnel: [w3273] -> w102
    tunnel: w102 -> [w3314]
    frame #0 {
      n2272 = while {
        stop <- w3266 continue-if-true
        n2273 = call "Close Video Capture.vi"() -> ("error code OUT"=w3268:i32)
        n2274 = Equal?(x=w3268, y=0) -> (x = y?=w3266:bool)
      }
      n2275 = local write "Stop All"(FALSE ("Stop All")) -> ()
    }
    frame #1 {
      n2276 = call "DMR_Init.vi"() -> ()  [unwired: 3 out]
    }
    frame #2 {
      # "Setting the destination format to Mono8 makes sure that the image can be displayed in the intensity plot."
      n2277 = call "DMR_GetDevice.vi"("search string IN"="DE019116701") -> ("device handle OUT"=w3291:i32)  [unwired: 4 in, 2 out]
      n2278 = call "DMR_OpenDevice.vi"("device handle IN"=w3291) -> ("driver handle OUT"=w3274:i32)  [unwired: 4 out]
      n2279 = call "DMR_FindList.vi"("flags IN"=u32 0 ("flags"), "list name IN"="" ("String"), "list type IN"=T32."camera descriptions", "driver handle IN"=w3274) -> ("list handle OUT"=w3277:i32)  [unwired: 2 out]
      n2280 = call "DMR_FindList.vi"("flags IN"=u32 0 ("flags"), "list name IN"="Base", "list type IN"=T32."setting", "driver handle IN"=w3274) -> ("list handle OUT"=w3275:i32)  [unwired: 2 out]
      n2281 = call "OBJ_GetHandle.vi"("object name IN"="VideoStandard", "list handle IN"=w3277) -> ("object handle OUT"=w3271:i32)  [unwired: 3 out]
      n2282 = call "OBJ_GetHandle.vi"("object name IN"="PixelFormat", "list handle IN"=w3275) -> ("object handle OUT"=w3285:i32)  [unwired: 3 out]
      n2283 = call "OBJ_SetS.vi"("value index IN"=0, "value IN"="NTSC M", "object handle IN"=w3271) -> ()  [unwired: 2 out]
      n2284 = call "OBJ_SetS.vi"("value index IN"=0, "value IN"="Mono8" ("value"), "object handle IN"=w3285) -> ()  [unwired: 2 out]
      n2285 = call "OBJ_GetHandle.vi"("object name IN"="VideoChannel", "list handle IN"=w3275) -> ("object handle OUT"=w3281:i32)  [unwired: 3 out]
      n2286 = while {
        tunnel: [w3296] -> w3273
        tunnel: w3274 -> [w3293]
        stop <- w3294 continue-if-true
        n2287 = call "DMR_ImageRequestSingle.vi"("request control IN"=0, "driver handle IN"=w3293) -> ("error code OUT"=w3295:i32, "driver handle OUT"=w3296:i32)  [unwired: 2 out]
        n2288 = Equal To 0?(x=w3295) -> (x = 0?=w3294:bool)
      }
      n2289 = call "OBJ_SetI.vi"("value index IN"=0, "value IN"=3 ("Video channel"), "object handle IN"=w3281) -> ()  [unwired: 2 out]
    }
    frame #3 {
      w3302 = T17 0 items=["Grayscale (U8)", "Grayscale (I16)", "Grayscale (SGL)", "Complex (CSG)", "RGB (U32)", "HSL (U32)", "RGB (U64)"] ("Image Type")
      w3310 = T17 0 items=["Grayscale (U8)", "Grayscale (I16)", "Grayscale (SGL)", "Complex (CSG)", "RGB (U32)", "HSL (U32)", "RGB (U64)"] ("Image Type")
      n2290 = for "Create Greyscale map" {
        N: 256 -> [_]
        tunnel: [w3316] -> w3299 mode=indexing
        workers-P: _ -> [_]
        i -> [w3319]
        n2291 = To Unsigned Byte Integer(number=w3319) -> (unsigned 8bit integer=w3315:u8)
        n2292 = Join Numbers(hi=w3315, lo=w3315) -> ((hi.lo)=w3318:u16)
        n2293 = Join Numbers(hi=w3315, lo=w3315) -> ((hi.lo)=w3317:u16)
        n2294 = Join Numbers(hi=w3318, lo=w3317) -> ((hi.lo)=w3316:u32)
      }
      n2295 = call "IMAQ Create"("Image Name"="Scaled video", "Image Type"=w3302) -> ("New Image"=w3301:T2)  [unwired: 2 in, 2 out]
      n2296 = call "IMAQ Create"("Image Name"="Main video", "Image Type"=w3310) -> ("New Image"=w3311:T2)  [unwired: 2 in, 2 out]
      n2297 = node-c288(0 ("Processor")) -> (w3309:T21)  [unwired: 3 out]
      n2298 = Initialize Array(u32 0 ("Window Number (0...15)"), 480 ("dimension size"), 640 ("dimension size")) -> (w3304:u32[][])
      n2299 = timed-loop {
        tunnel: w3314 -> [w3336]
        tunnel: [w3335] -> w3313
        tunnel: w3311 -> [w3334]
        timing: w3309 -> [_]
        timing-out: [_] -> w3308
        tunnel: w3304 -> [w3323]
        tunnel: w3301 -> [w3321]
        tunnel: w3299 -> [w3320]
        stop <- w3322 stop-if-true
        # "This block performs the \nactual image capture."
        n2300 = node-c288() -> ()  [unwired: 2 out]
        n2301 = local read "Stop All"() -> (w3322:bool)
        n2302 = Reciprocal(x="Video Capture Rate (Hz)") -> (1/x=w3326:dbl)
        n2303 = Multiply(x=w3326, y=1000.0) -> (x*y=w3324:dbl)
        n2304 = call "DMR_ImageRequestWaitFor.vi"("queue number IN"=0, "timeout(ms) IN"=500, "driver handle IN"=w3336) -> ("error code OUT"=w3340:i32, "request number OUT"=w3337:i32, "driver handle OUT"=w3338:i32)
        n2305 = feedback #1(T33 refnum ("Avi Refnum")) -> (w3328:T33)
        n2306 = case shown="True" "New Video File" {
          tunnel: [T33 refnum ("Avi Refnum") w3357] -> w3330
          tunnel: [FALSE TRUE] -> w3331
          tunnel: w3328 -> [_ w3353]
          frame False {
          }
          frame True {
            n2307 = call "Create new save file.vi"("Ext"=".avi" ("string"), "Index In"="Video Index") -> ("Path Out"=w3349:path, "Index Out"=w3350:dbl)  [unwired: 1 in]
            "Path Out" <- w3349
            n2308 = Not Equal?(x=w3353, y=T33 refnum ("Avi Refnum")) -> (x != y?=w3354:bool)
            n2309 = Increment(x=w3350) -> (x+1=w3359:dbl)
            n2310 = case shown="True" w3354 {
              tunnel: w3353 -> [_ w3360]
              frame False {
              }
              frame True {
                n2311 = call "IMAQ AVI Close"("Avi Refnum"=w3360) -> ()  [unwired: 1 in, 10 out]
              }
            }
            n2312 = local write "Video Index"(w3359) -> ()
            n2313 = call "IMAQ AVI Create"("Frames Per Second"=u32 30, "AVI Path"=w3349) -> ("Avi Refnum"=w3357:T33)  [unwired: 5 in, 4 out]
          }
        }
        n2314 = Equal To 0?(x=w3340) -> (x = 0?=w3339:bool)
        n2315 = Select(t=w3330, s=w3331, f=w3328) -> (s? t:f=w3329:T33)
        n2316 = feedback-in #1(w3329) -> ()
        n2317 = case shown="True" w3339 {
          tunnel: w3338 -> [w3361 w3388]
          tunnel: w3337 -> [_ w3387]
          tunnel: [w3361 w3384] -> w3335
          tunnel: w3334 -> [_ w3365]
          tunnel: w3323 -> [_ w3372]
          tunnel: w3329 -> [_ w3370]
          tunnel: w3321 -> [_ w3366]
          tunnel: w3320 -> [_ w3367]
          frame False {
          }
          frame True {
            w3378 = u32 0 ("X-offset IN")
            n2318 = call "DMR_GetImageRequestBufferData.vi"("driver handle IN"=w3388, "request number IN"=w3387) -> ("width OUT"=w3377:i32, "height OUT"=w3376:i32, "driver handle OUT"=w3383:i32, "request number OUT"=w3382:i32, "bytes per pixel OUT"=w3379:i32)  [unwired: 13 out]
            n2319 = call "DMR_GetImageRequestBufferImageData.vi"("driver handle IN"=w3383, "request number IN"=w3382, "bytes per pixel IN"=w3379, "X-offset IN"=w3378, "Y-offset IN"=w3378, "height IN"=w3376, "width IN"=w3377) -> ("driver handle OUT"=w3381:u32, "request number OUT"=w3380:u32, "image OUT"=w3373:u32[][])  [unwired: 10 out]
            n2320 = call "DMR_ImageRequestUnlock.vi"("request number IN"=w3380, "driver handle IN"=w3381) -> ("driver handle OUT"=w3386:i32)  [unwired: 1 in, 2 out]
            n2321 = case shown="True" "Averaging" {
              tunnel: w3373 -> [w3429 w3434]
              tunnel: [w3429 w3433] -> w3369
              tunnel: w3372 -> [_ w3431]
              frame False {
              }
              frame True {
                (unwired) 1
                w3439 = 1
                n2322 = feedback #2(w3431) -> (w3430:u32[][])
                n2323 = Add(x=w3434, y=w3430) -> (x+y=w3435:u32[][])
                n2324 = Select(t=w3431, s="Reset Averaging", f=w3435) -> (s? t:f=w3437:u32[][])
                n2325 = feedback-in #2(w3437) -> ()
                n2326 = feedback #3(w3439) -> (w3432:i32)
                n2327 = Divide(x=w3435, y=w3432) -> (x/y=w3436:dbl[][])
                n2328 = Increment(x=w3432) -> (x+1=w3440:i32)
                n2329 = To Unsigned Long Integer(number=w3436) -> (unsigned 32bit integer=w3433:u32[][])
                n2330 = Select(t=w3439, s="Reset Averaging", f=w3440) -> (s? t:f=w3438:i32)
                n2331 = feedback-in #3(w3438) -> ()
              }
            }
            n2332 = call "DMR_ImageRequestSingle.vi"("request control IN"=0, "driver handle IN"=w3386) -> ("driver handle OUT"=w3384:i32)  [unwired: 3 out]
            n2333 = disable-structure shown="Disabled" {
              disable-tunnel: w3369 -> [w3406 _]
              disable-tunnel: w3366 -> [w3405 _]
              frame Disabled {
                n2334 = To Double Precision Float(number=w3406) -> (double precision float=w3404:dbl[][])
                n2335 = In Range and Coerce(upper limit="Intensity Upper", x=w3404, lower limit="Intensity Lower") -> (coerced(x)=w3403:dbl[][])  [unwired: 1 out]
                n2336 = Subtract(x="Intensity Upper", y="Intensity Lower") -> (x-y=w3400:dbl)
                n2337 = Subtract(x=w3403, y="Intensity Lower") -> (x-y=w3401:dbl[][])
                n2338 = Divide(x=w3401, y=w3400) -> (x/y=w3402:dbl[][])
                n2339 = Multiply(x=255.0, y=w3402) -> (x*y=w3398:dbl[][])
                n2340 = To Unsigned Byte Integer(number=w3398) -> (unsigned 8bit integer=w3407:u8[][])
                n2341 = call "IMAQ ArrayToImage"("Image Pixels (U8)"=w3407, "Image"=w3405) -> ("Image Out"=w3394:T2)  [unwired: 4 in, 5 out]
                n2342 = First Call?() -> (First Call?: T/F=w3395:bool)
                n2343 = case shown="True" w3395 {
                  tunnel: w3394 -> [w3408 w3419]
                  frame False {
                    n2344 = flat-sequence {
                      tunnel: w3408 -> [w3414]
                      frame #0 {
                        w3411 = FALSE ("Get/Set Status? (Set)")
                        w3410 = 0 ("Window Number (0...15)")
                        n2345 = call "IMAQ WindSize"("Get/Set Status? (Set)"=w3411, "Window Number"=w3410) -> ("Width & Height out"=→"Window Size":cluster{"Width":i32, "Height":i32})  [unwired: 4 in, 2 out]
                        n2346 = call "IMAQ WindMove"("Window Number (0...15)"=w3410, "Get/Set Status? (Set)"=w3411) -> ("Coordinates (screen)"=→"Window Position":cluster{"X Position":i32, "Y Position":i32})  [unwired: 3 in, 1 out]
                        n2347 = call "IMAQ WindDraw"("Resize to Image Size? (Y)"=FALSE, "Window Number (0...15)"=w3410, "Image"=w3414) -> ()  [unwired: 7 in, 2 out]
                      }
                      frame #1 {
                        n2348 = call "IMAQ WindZoom 2"("Center Point"="Center Point", "Zoom to Fit? (False)"=FALSE, "Zoom Factor"="Zoom Factor") -> ()  [unwired: 5 in, 4 out]
                      }
                    }
                  }
                  frame True {
                    n2349 = flat-sequence {
                      tunnel: w3419 -> [w3422]
                      tunnel: [w3420] -> w3418
                      tunnel: w3418 -> [w3424]
                      frame #0 {
                        w3421 = TRUE ("Resize to Image Size? (Y)")
                        w3420 = 0 ("Window Number (0...15)")
                        n2350 = call "IMAQ WindNonTearing"("Window Number"=w3420, "NonTearing? (True)"=w3421) -> ()  [unwired: 8 in, 2 out]
                        n2351 = call "IMAQ WindDraw"("Resize to Image Size? (Y)"=w3421, "Window Number (0...15)"=w3420, "Image"=w3422) -> ()  [unwired: 7 in, 2 out]
                      }
                      frame #1 {
                        n2352 = call "IMAQ WindSize"("Scrollbars? (N)"=FALSE, "Width & Height"="Initial Window Size", "Window Number"=w3424) -> ()  [unwired: 3 in, 3 out]
                        n2353 = call "IMAQ WindMove"("Window Number (0...15)"=w3424, "Coordinates (screen)"="Initial Window Position") -> ()  [unwired: 3 in, 2 out]
                      }
                    }
                  }
                }
              }
              frame Enabled {
              }
            }
            n2354 = To Unsigned Byte Integer(number=w3369) -> (unsigned 8bit integer=w3368:u8[][])
            n2355 = call "IMAQ ArrayToImage"("Image Pixels (U8)"=w3368, "Image"=w3365) -> ("Image Out"=w3363:T2)  [unwired: 4 in, 5 out]
            n2356 = case shown="True" "Save Video" {
              tunnel: w3370 -> [_ w3428]
              tunnel: w3363 -> [_ w3427]
              frame False {
              }
              frame True {
                n2357 = call "IMAQ AVI Write Frame"("Image"=w3427, "Avi Refnum"=w3428) -> ()  [unwired: 2 in, 8 out]
              }
            }
            n2358 = case shown="True" "Save Image" {
              tunnel: w3368 -> [_ w3443]
              tunnel: w3367 -> [_ w3442]
              frame False {
              }
              frame True {
                n2359 = call <vilib>:"Flatten Pixmap.vi"("colors"=w3442, "8-bit pixmap"=w3443) -> ("image data"=w3449:T34)  [unwired: 4 in, 5 out]
